vi "Controller Settings Dialog.vi"(8 "error in (no error)":errorcluster, 11 "Settings in":T1={"Logging Configuration"={"Log File Base Path"=path "", "Samples to Save"=0, "Acquisition Sample Rate"=0.0, "SamplesPerChannel"=0, "FFT - Block Size"=0, "FFT - NumberOfAverages"=0, "Trigger - Time"=0, "Trigger - Threshold"=0.0, "Trigger - Channel"=0, "Enable Time Trigger"=FALSE, "Enable Threshold Trigger"=FALSE, "Always Log"=FALSE, "Enable Filter"=FALSE, "FilesRefs"={"TimeDomainTDMSRef"=refnum, "FreuencyDomainTDMSRef"=refnum, "TXT-FileRef"=refnum}, "OutputFileFormat"=enum."TXT", "ActualBlockSize"=0, "HasBeenTriggeredAlready"=FALSE, "Start Time"=timestamp(0 s since 1904-01-01)}, "Hardware Configuration"={"Accel-ai0"=FALSE, "Maximum Input"=0.0, "Minimum Input"=0.0, "HW Sample Rate"=0.0, "SW Sample Rate"=0.0, "Number of Samples"=0, "Accel-ai1"=FALSE, "DAQmx Task"="", "Low Pass Filter"={"Upper Cutoff"=350.0, "Lower Cutoff"=350.0, "Order"=350}}} {"Hardware Configuration"."Low Pass Filter"."Order" min=0 max=10 step=1}) -> (0 "error out":errorcluster, 1 "Cancelled?":bool=TRUE, 2 "UI Refresh Needed?":bool, 3 "Settings Out":T1={"Logging Configuration"={"Log File Base Path"=path "", "Samples to Save"=0, "Acquisition Sample Rate"=0.0, "SamplesPerChannel"=0, "FFT - Block Size"=0, "FFT - NumberOfAverages"=0, "Trigger - Time"=0, "Trigger - Threshold"=0.0, "Trigger - Channel"=0, "Enable Time Trigger"=FALSE, "Enable Threshold Trigger"=FALSE, "Always Log"=FALSE, "Enable Filter"=FALSE, "FilesRefs"={"TimeDomainTDMSRef"=refnum, "FreuencyDomainTDMSRef"=refnum, "TXT-FileRef"=refnum}, "OutputFileFormat"=enum."TXT", "ActualBlockSize"=0, "HasBeenTriggeredAlready"=FALSE, "Start Time"=timestamp(0 s since 1904-01-01)}, "Hardware Configuration"={"Accel-ai0"=FALSE, "Maximum Input"=0.0, "Minimum Input"=0.0, "HW Sample Rate"=0.0, "SW Sample Rate"=0.0, "Number of Samples"=0, "Accel-ai1"=FALSE, "DAQmx Task"="", "Low Pass Filter"={"Upper Cutoff"=350.0, "Lower Cutoff"=350.0, "Order"=350}}} {"Hardware Configuration"."Low Pass Filter"."Order" min=0 max=10 step=1})   [LabVIEW 2022 SP3, in "Settings.lvlib"]
doc: "Dialog for selecting user specified settings."
uses:
  Settings.lvlib
  <resource>/objmgr/daqmx.rc
  <vilib>/Utility/xml.llb/Write to XML File(string).vi
  Logging/Logging Configuration.ctl
  Logging/Logging.lvlib
  Settings.ctl
  FiniteMeasurement-DAQmx/controls/Hardware Configuration.ctl
  Acquisition/Acquisition.lvlib
  support/TDMS-Refs.ctl
  AcquisitionFilter.ctl
panel:
  out "Frequency Delta(Hz)":dbl
  in  "Logging Configuration.Enable Filter":bool
  in  "Upper Cutoff":dbl
  in  "Lower Cutoff":dbl
  in  "Order":i32
  in  "Number of FFT Averages":i32=5
  in  "Block Size":u32 max=10240 step=10
  in  "Accelerometer AI-1":bool
  in  "Accelerometer AI-0":bool=TRUE
  in  "Log when triggered":bool
  in  "Trigger Channel":u32
  in  "Samples to Log":u32=206000 min=1
  in  "Trigger Threshold (V)":dbl=2.0
  in  "Trigger Time (s)":u32=1
  in  "Enable Threshold Trigger (V):":bool
  in  "Enable Time Trigger (s):":bool
  in  "Always Log":bool
  in  "Sample Rate":dbl=41200.0
  in  "Minimum Input":dbl=-5.0
  in  "Maximum Input":dbl=5.0
  in  "Log Base Path":path=path "C:/Users/LAV-UFSC-2023/Documents/LAV-TCC/Dados-Experimentos/Dados-Bancada-LABVIEW/teste.txt"
  in  "Cancel Button":bool
  in  "OK Button":bool
  # "Acquisition"
  # "LowPassFilter"
  # "Non visible portion of dialog (needed for connector pane)."
  # "Trigger"
  # "Logging"
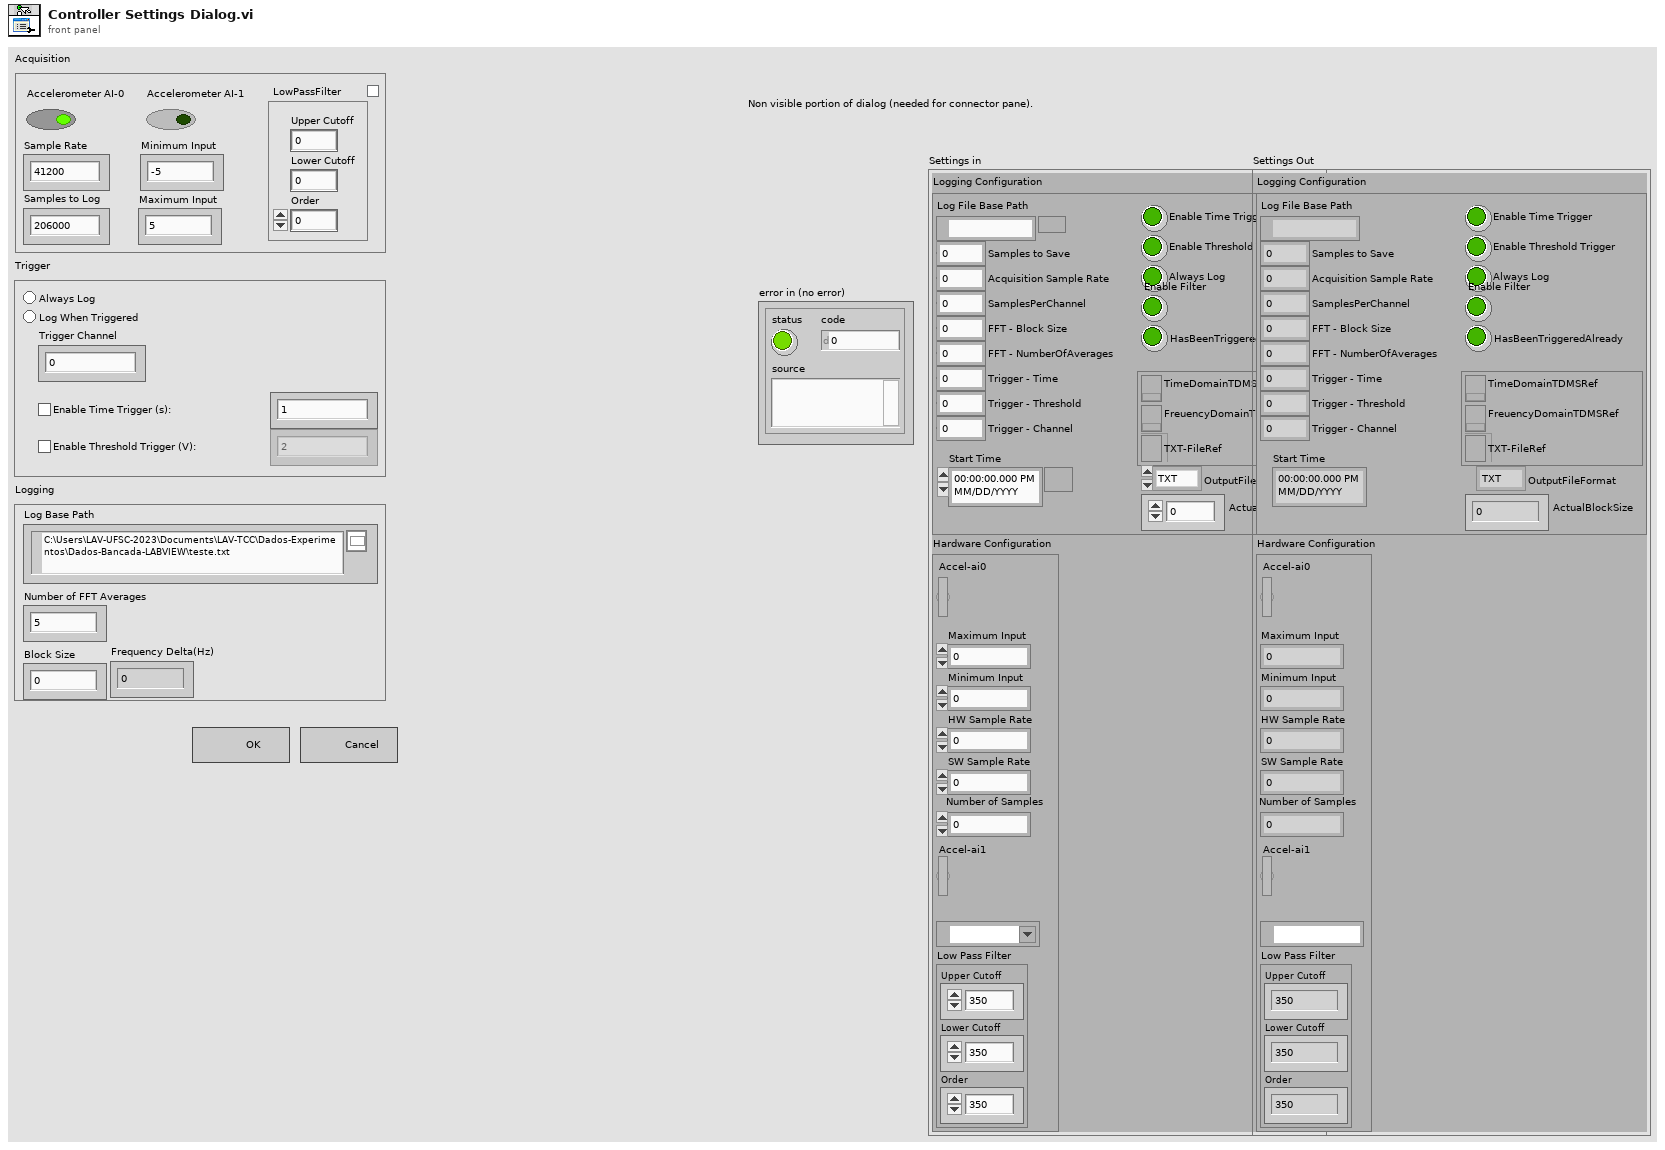
[diagram p1: front panel]
types:
  T1 = typedef "Settings.lvlib/Settings.ctl" = cluster{"Logging Configuration":T2, "Hardware Configuration":T4}
  T2 = typedef "Logging.lvlib/Logging Configuration.ctl" = cluster{"Log File Base Path":path, "Samples to Save":u32, "Acquisition Sample Rate":dbl, "SamplesPerChannel":u32, "FFT - Block Size":u32, "FFT - NumberOfAverages":i32, "Trigger - Time":i32, "Trigger - Threshold":dbl, "Trigger - Channel":i32, "Enable Time Trigger":bool, "Enable Threshold Trigger":bool, "Always Log":bool, "Enable Filter":bool, "FilesRefs":T3, "OutputFileFormat":enum16{"TXT", "TDMS"}, "ActualBlockSize":i32, "HasBeenTriggeredAlready":bool, "Start Time":timestamp}
  T3 = typedef "TDMS-Refs.ctl" = cluster{"TimeDomainTDMSRef":refnum<k34>, "FreuencyDomainTDMSRef":refnum<k34>, "TXT-FileRef":refnum<file>}
  T4 = typedef "Acquisition.lvlib/Hardware Configuration.ctl" = cluster{"Accel-ai0":bool, "Maximum Input":dbl, "Minimum Input":dbl, "HW Sample Rate":dbl, "SW Sample Rate":dbl, "Number of Samples":i32, "Accel-ai1":bool, "DAQmx Task":refnum<k21>, "Low Pass Filter":T5}
  T5 = typedef "Acquisition.lvlib/AcquisitionFilter.ctl" = cluster{"Upper Cutoff":dbl, "Lower Cutoff":dbl, "Order":i32}
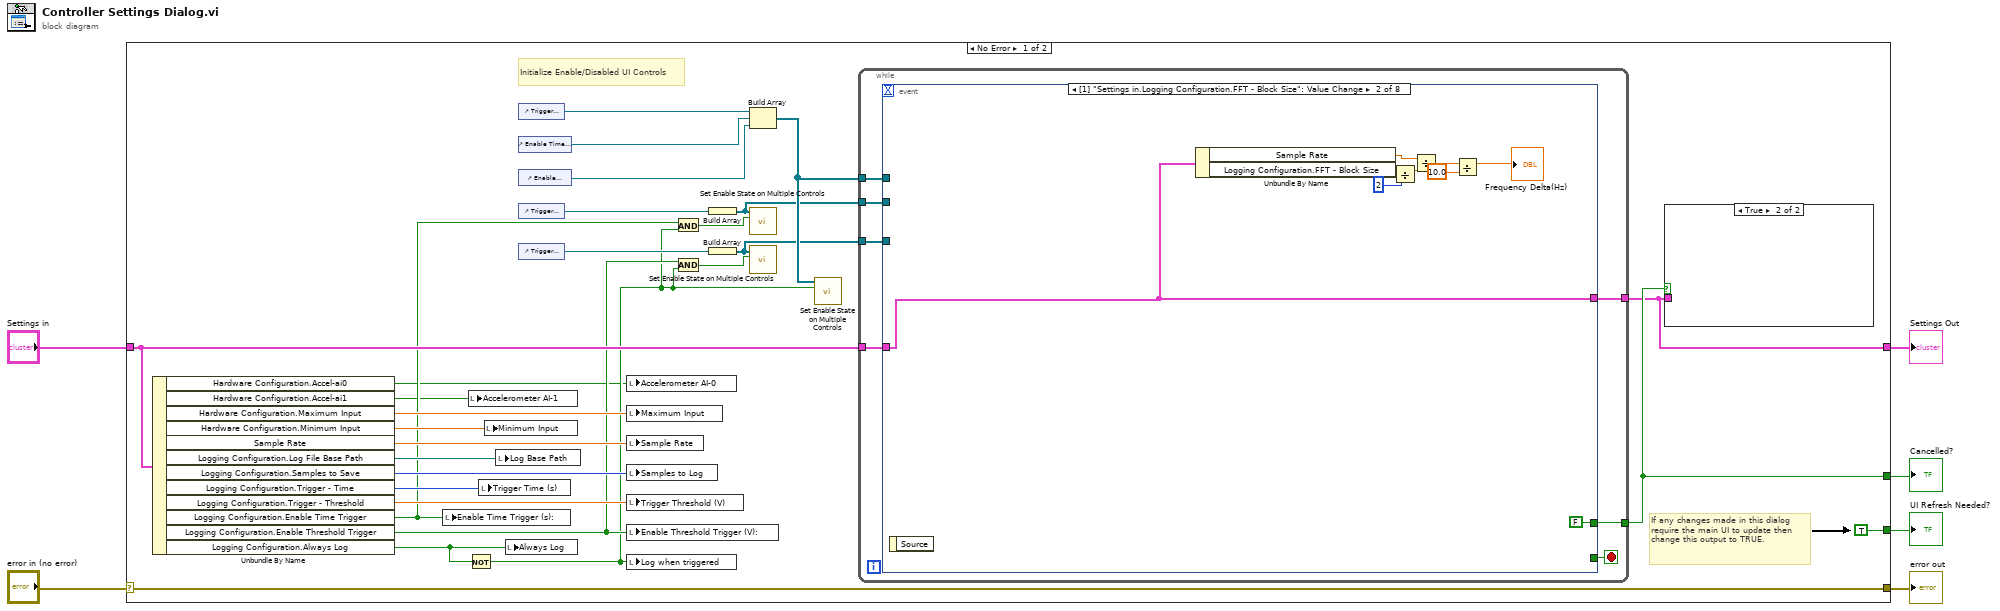
[diagram p0: block diagram]
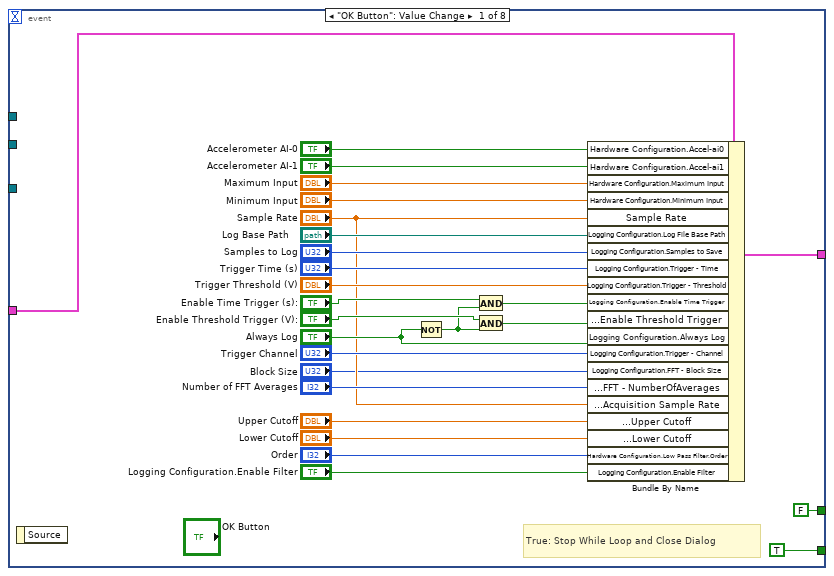
[diagram p2: hidden frame]
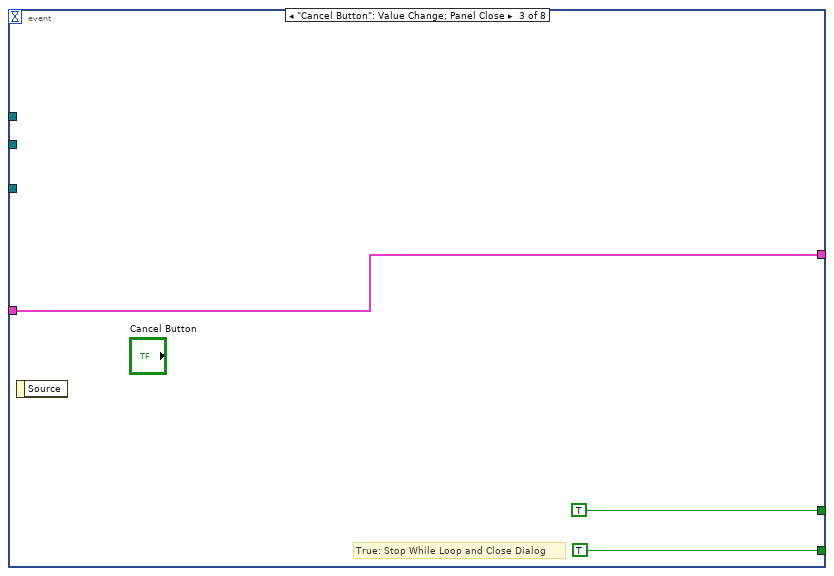
[diagram p3: hidden frame]
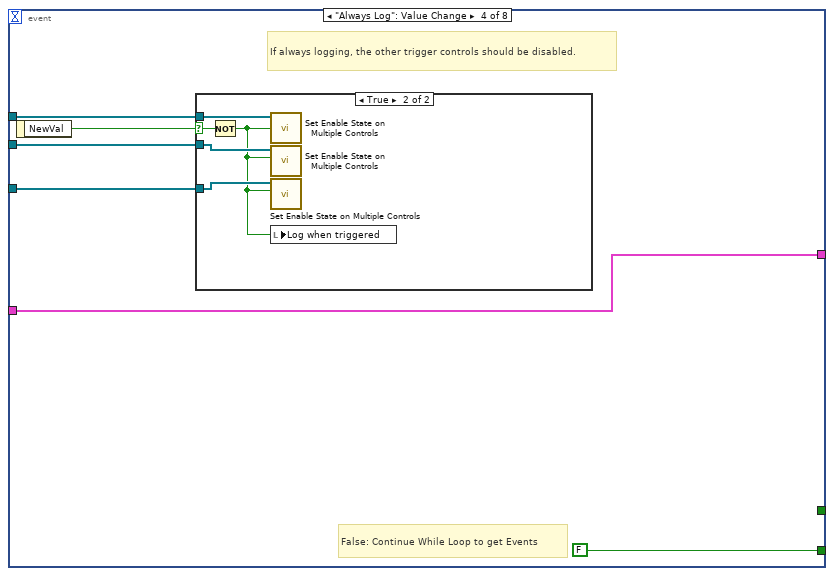
[diagram p4: hidden frame]
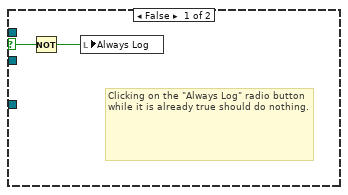
[diagram p5: hidden frame]
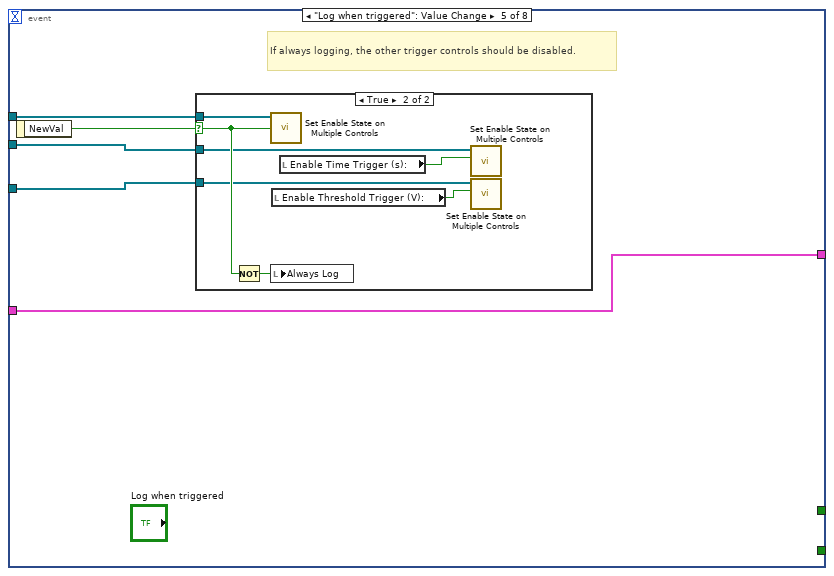
[diagram p6: hidden frame]
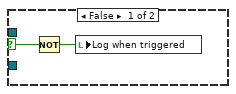
[diagram p7: hidden frame]
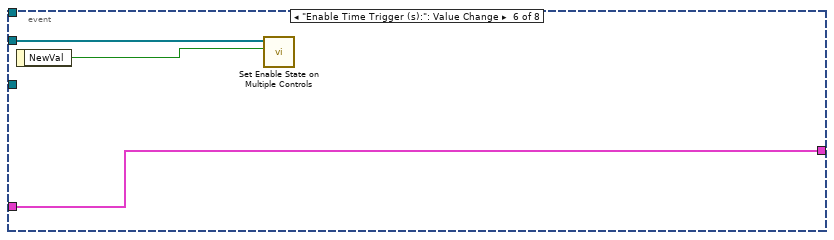
[diagram p8: hidden frame]
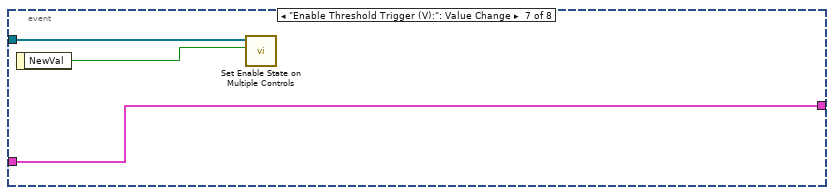
[diagram p9: hidden frame]
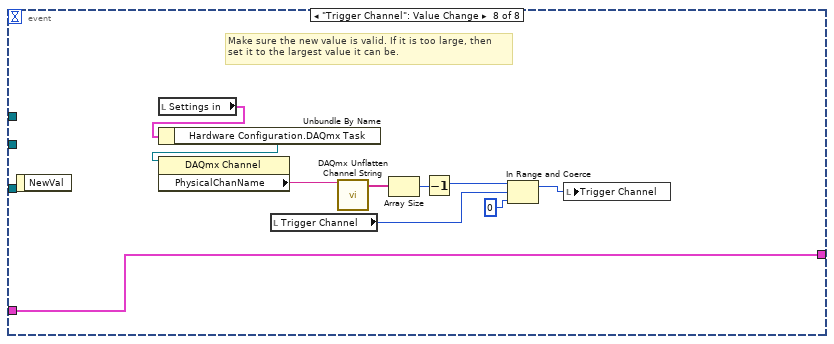
[diagram p10: hidden frame]
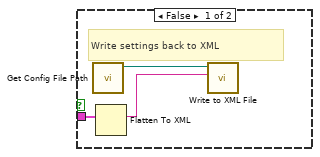
[diagram p11: hidden frame]
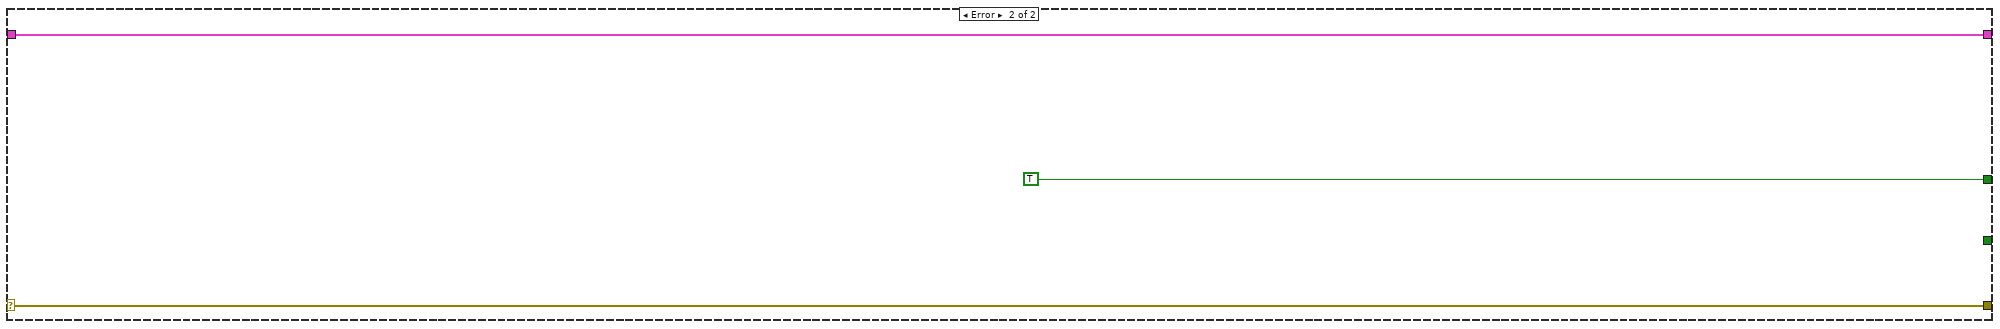
[diagram p12: hidden frame]
diagram:
  n1 = case shown="No Error" "error in (no error)" {
    selector: "error in (no error)" -> [w34 w128]
    tunnel: [w34 w128] -> w6
    tunnel: "Settings in" -> [w21 w127]
    tunnel: [w31 w127] -> w5
    tunnel: [TRUE ("UI Refresh Needed?") _] -> w4
    tunnel: [w32 TRUE ("UI Refresh Needed?")] -> w3
    frame No Error {
      # "Initialize Enable/Disabled UI Controls"
      # "If any changes made in this dialog require the main UI to update then change this output to TRUE."
      n2 = Unbundle By Name(w21) -> ("Hardware Configuration.Accel-ai0"=w7:bool, "Hardware Configuration.Accel-ai1"=w8:bool, "Hardware Configuration.Maximum Input"=w28:dbl, "Hardware Configuration.Minimum Input"=w29:dbl, "Sample Rate"=w30:dbl, "Logging Configuration.Log File Base Path"=w27:path, "Logging Configuration.Samples to Save"=w26:u32, "Logging Configuration.Trigger - Time"=w25:i32, "Logging Configuration.Trigger - Threshold"=w24:dbl, "Logging Configuration.Enable Time Trigger"=w13:bool, "Logging Configuration.Enable Threshold Trigger"=w12:bool, "Logging Configuration.Always Log"=w23:bool)
      n3 = local write "Enable Time Trigger (s):"(w13) -> ()
      n4 = Not(x=w23) -> (.not. x?=w9:bool)
      n5 = local write "Accelerometer AI-1"(w8) -> ()
      n6 = local write "Trigger Time (s)"(w25) -> ()
      n7 = local write "Minimum Input"(w29) -> ()
      n8 = local write "Log Base Path"(w27) -> ()
      n9 = local write "Always Log"(w23) -> ()
      n10 = control-ref of="Trigger Channel"() -> (w20:refnum<vi>)
      n11 = control-ref of="Enable Time Trigger (s):"() -> (w19:refnum<vi>)
      n12 = control-ref of="Enable Threshold Trigger (V):"() -> (w18:refnum<vi>)
      n13 = control-ref of="Trigger Time (s)"() -> (w17:refnum<vi>)
      n14 = control-ref of="Trigger Threshold (V)"() -> (w16:refnum<vi>)
      n15 = local write "Accelerometer AI-0"(w7) -> ()
      n16 = local write "Maximum Input"(w28) -> ()
      n17 = local write "Sample Rate"(w30) -> ()
      n18 = local write "Samples to Log"(w26) -> ()
      n19 = local write "Trigger Threshold (V)"(w24) -> ()
      n20 = local write "Enable Threshold Trigger (V):"(w12) -> ()
      n21 = local write "Log when triggered"(w9) -> ()
      n22 = And(x=w13, y=w9) -> (x .and. y?=w15:bool)
      n23 = And(x=w12, y=w9) -> (x .and. y?=w14:bool)
      n24 = Build Array(w17) -> (w11:refnum<vi>[])
      n25 = Build Array(w16) -> (w10:refnum<vi>[])
      n26 = Build Array(w20, w19, w18) -> (w22:refnum<vi>[])
      n27 = call "Set Enable State on Multiple Controls.vi"("Enable?"=w15, "Controls"=w11) -> ()  [unwired: 10 in]
      n28 = call "Set Enable State on Multiple Controls.vi"("Enable?"=w14, "Controls"=w10) -> ()  [unwired: 10 in]
      n29 = call "Set Enable State on Multiple Controls.vi"("Enable?"=w9, "Controls"=w22) -> ()  [unwired: 10 in]
      n30 = while {
        tunnel: [w41] -> w32
        tunnel: [w40] -> w31
        tunnel: w21 -> [w39]
        tunnel: w22 -> [w37]
        tunnel: w11 -> [w36]
        tunnel: w10 -> [w35]
        stop <- w38 stop-if-true
        n31 = event shown="[1] \"Settings in.Logging Configuration.FFT - Block Size\": Value Change" {
          selector: _ -> [_ _ _ _ _ _ _ _]
          dyn-events: _ -> [_ _ _ _ _ _ _ _]
          timeout: _ -> [_ _ _ _ _ _ _ _]
          tunnel: [w65 w76 w79 w85 w97 w109 w112 w122] -> w40
          tunnel: w39 -> [w64 w76 w79 w85 w97 w109 w112 w122]
          tunnel: [FALSE ("UI Refresh Needed?") FALSE ("UI Refresh Needed?") TRUE ("UI Refresh Needed?") _ _ _ _ _] -> w41
          tunnel: [TRUE _ TRUE FALSE _ _ _ _] -> w38
          tunnel: w37 -> [_ _ _ w83 w96 _ _ _]
          tunnel: w36 -> [_ _ _ w81 w94 w108 _ _]
          tunnel: w35 -> [_ _ _ w80 w93 _ w111 _]
          event "OK Button": Value Change {
            # "True: Stop While Loop and Close Dialog"
            n32 = event-data() -> ()  [unwired: 1 in, 1 out]
            n33 = Not(x="Always Log") -> (.not. x?=w51:bool)
            n34 = And(x="Enable Time Trigger (s):", y=w51) -> (x .and. y?=w52:bool)
            n35 = And(x="Enable Threshold Trigger (V):", y=w51) -> (x .and. y?=w54:bool)
            n36 = Bundle By Name(cluster=w64, "Hardware Configuration.Accel-ai0"="Accelerometer AI-0", "Hardware Configuration.Accel-ai1"="Accelerometer AI-1", "Hardware Configuration.Maximum Input"="Maximum Input", "Hardware Configuration.Minimum Input"="Minimum Input", "Sample Rate"="Sample Rate", "Logging Configuration.Log File Base Path"="Log Base Path", "Logging Configuration.Samples to Save"="Samples to Log", "Logging Configuration.Trigger - Time"="Trigger Time (s)", "Logging Configuration.Trigger - Threshold"="Trigger Threshold (V)", "Logging Configuration.Enable Time Trigger"=w52, "Logging Configuration.Enable Threshold Trigger"=w54, "Logging Configuration.Always Log"="Always Log", "Logging Configuration.Trigger - Channel"="Trigger Channel", "Logging Configuration.FFT - Block Size"="Block Size", "Logging Configuration.FFT - NumberOfAverages"="Number of FFT Averages", "Logging Configuration.Acquisition Sample Rate"="Sample Rate", "Hardware Configuration.Low Pass Filter.Upper Cutoff"="Upper Cutoff", "Hardware Configuration.Low Pass Filter.Lower Cutoff"="Lower Cutoff", "Hardware Configuration.Low Pass Filter.Order"="Order", "Logging Configuration.Enable Filter"="Logging Configuration.Enable Filter") -> (w65:T1)
          }
          event Value Change {
            n37 = event-data() -> ()  [unwired: 1 in, 1 out]
            n38 = Unbundle By Name(w76) -> ("Sample Rate"=w75:dbl, "Logging Configuration.FFT - Block Size"=w74:u32)
            n39 = Divide(x=w74, y=u32 2) -> (x/y=w70:dbl)
            n40 = Divide(x=w75, y=w70) -> (x/y=w73:dbl)
            n41 = Divide(x=w73, y=10.0) -> (x/y=→"Frequency Delta(Hz)":dbl)
          }
          event "Cancel Button": Value Change; Panel Close {
            # "True: Stop While Loop and Close Dialog"
            n42 = event-data() -> ()  [unwired: 1 in, 1 out]
          }
          event "Always Log": Value Change {
            # "False: Continue While Loop to get Events"
            # "If always logging, the other trigger controls should be disabled."
            n43 = event-data() -> ("NewVal"=w82:bool)  [unwired: 1 in]
            n44 = case shown="True" w82 {
              selector: w82 -> [w87 w92]
              tunnel: w83 -> [_ w91]
              tunnel: w81 -> [_ w90]
              tunnel: w80 -> [_ w89]
              frame False {
                # "Clicking on the \"Always Log\" radio button while it is already true should do nothing."
                n45 = Not(x=w87) -> (.not. x?=w86:bool)
                n46 = local write "Always Log"(w86) -> ()
              }
              frame True {
                n47 = Not(x=w92) -> (.not. x?=w88:bool)
                n48 = call "Set Enable State on Multiple Controls.vi"("Enable?"=w88, "Controls"=w91) -> ()  [unwired: 10 in]
                n49 = call "Set Enable State on Multiple Controls.vi"("Enable?"=w88, "Controls"=w90) -> ()  [unwired: 10 in]
                n50 = call "Set Enable State on Multiple Controls.vi"("Enable?"=w88, "Controls"=w89) -> ()  [unwired: 10 in]
                n51 = local write "Log when triggered"(w88) -> ()
              }
            }
          }
          event "Log when triggered": Value Change {
            # "If always logging, the other trigger controls should be disabled."
            n52 = event-data() -> ("NewVal"=w95:bool)  [unwired: 1 in]
            n53 = case shown="True" w95 {
              selector: w95 -> [w99 w105]
              tunnel: w96 -> [_ w106]
              tunnel: w94 -> [_ w103]
              tunnel: w93 -> [_ w102]
              frame False {
                n54 = Not(x=w99) -> (.not. x?=w98:bool)
                n55 = local write "Log when triggered"(w98) -> ()
              }
              frame True {
                n56 = Not(x=w105) -> (.not. x?=w104:bool)
                n57 = call "Set Enable State on Multiple Controls.vi"("Enable?"=w105, "Controls"=w106) -> ()  [unwired: 10 in]
                n58 = local write "Always Log"(w104) -> ()
                n59 = local read "Enable Threshold Trigger (V):"() -> (w101:bool)
                n60 = local read "Enable Time Trigger (s):"() -> (w100:bool)
                n61 = call "Set Enable State on Multiple Controls.vi"("Enable?"=w100, "Controls"=w103) -> ()  [unwired: 10 in]
                n62 = call "Set Enable State on Multiple Controls.vi"("Enable?"=w101, "Controls"=w102) -> ()  [unwired: 10 in]
              }
            }
          }
          event "Enable Time Trigger (s):": Value Change {
            n63 = event-data() -> ("NewVal"=w107:bool)  [unwired: 1 in]
            n64 = call "Set Enable State on Multiple Controls.vi"("Enable?"=w107, "Controls"=w108) -> ()  [unwired: 10 in]
          }
          event "Enable Threshold Trigger (V):": Value Change {
            n65 = event-data() -> ("NewVal"=w110:bool)  [unwired: 1 in]
            n66 = call "Set Enable State on Multiple Controls.vi"("Enable?"=w110, "Controls"=w111) -> ()  [unwired: 10 in]
          }
          event "Trigger Channel": Value Change {
            # "Make sure the new value is valid. If it is too large, then\nset it to the largest value it can be."
            n67 = event-data() -> ()  [unwired: 1 in, 1 out]
            n68 = local read "Settings in"() -> (w115:T1)
            n69 = Unbundle By Name(w115) -> ("Hardware Configuration.DAQmx Task"=w114:refnum<k21>)
            n70 = property class="DAQmx Channel"(reference=w114) -> ("PhysicalChanName"=w113:tag)  [unwired: 1 in, 2 out]
            n71 = local read "Trigger Channel"() -> (w116:u32)
            n72 = call <vilib>:"DAQmx Unflatten Channel String.vi"("names in"=w113) -> ("names out"=w121:string[])  [unwired: 13 in, 1 out]
            n73 = Array Size(array=w121) -> (size(s)=w120:i32)
            n74 = Decrement(x=w120) -> (x-1=w119:i32)
            n75 = In Range and Coerce(upper limit=w119, x=w116, lower limit=u32 0) -> (coerced(x)=w117:u32)  [unwired: 1 out]
            n76 = local write "Trigger Channel"(w117) -> ()
          }
        }
      }
      n77 = case shown="True" w32 {
        tunnel: w31 -> [w124 _]
        frame False {
          # "Write settings back to XML"
          n78 = call "Get Config File Path.vi"() -> ("XML File Path"=w125:path)  [unwired: 10 in, 1 out]
          n79 = Flatten To XML(6:w124) -> (2:w123:string)
          n80 = call-poly <vilib>:"Write to XML File.vi"("XML Input"=w123, "XML File Path"=w125) -> ()  [unwired: 7 in, 3 out]
        }
        frame True {
        }
      }
    }
    frame Error {
    }
  }
  "UI Refresh Needed?" <- w4
  "error out" <- w6
  "Cancelled?" <- w3
  "Settings Out" <- w5
